vi "On Segmented Log Complete.vi"(8 "error in (no error)":errorcluster, 11 "File Open Event Registrations in":T1[](array[typedef])) -> (0 "error out":errorcluster, 3 "File Open Event Registrations out":T1[](array[typedef]))   [LabVIEW 2015, in "Waveform Data Logger Engine.lvlib" / "Segmented Log.lvclass"]
uses:
  Segmented Log.lvclass
  Segmented Log Complete Event Registration.ctl
  Segmented Log Complete Event Data.ctl
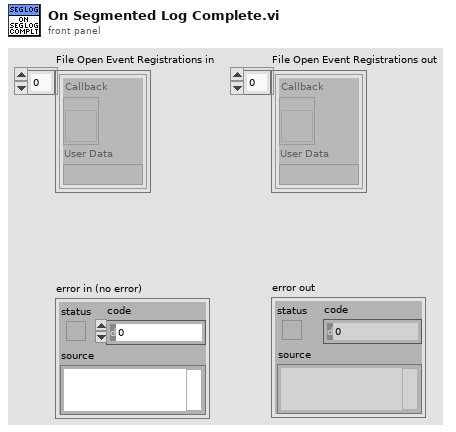
[diagram p1: front panel]
types:
  T1 = typedef "Waveform Data Logger Engine.lvlib/Segmented Log.lvclass/Segmented Log Complete Event Registration.ctl" = cluster{"Callback":refnum<vi>, "User Data":variant}
  T2 = typedef "Waveform Data Logger Engine.lvlib/Segmented Log.lvclass/Segmented Log Complete Event Data.ctl" = cluster{"User Data":variant}
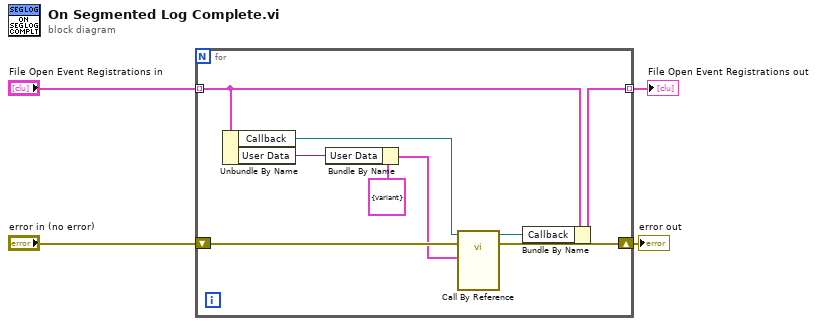
[diagram p0: block diagram]
diagram:
  n1 = for {
    tunnel: "File Open Event Registrations in" -> [w9] mode=indexing
    shift-right: [w10] -> w2
    shift-left: "error in (no error)" -> [w13]
    tunnel: [w8] -> w1 mode=indexing
    n2 = Unbundle By Name(w9) -> ("Callback"=w5:refnum<vi>, "User Data"=w11:variant)
    n3 = Bundle By Name(cluster=T2 {"User Data"=variant} ("Segmented Log Complete Event Data"), "User Data"=w11) -> (w6:T2)
    n4 = call-by-ref "?"(reference=w5, error in=w13, "Segmented Log Complete Event Data"=w6) -> (reference out=w7:refnum<vi>, error out=w10:errorcluster)  [unwired: 11 in]
    n5 = Bundle By Name(cluster=w9, "Callback"=w7) -> (w8:T1)
  }
  "error out" <- w2
  "File Open Event Registrations out" <- w1
